vi "Sensirion SHT25 - VISA soft reset.vi"(8 "Error In":errorcluster, 11 "VISA in":refnum<visa-resource-name>) -> (0 "Error Out":errorcluster, 1 "readback":string, 3 "VISA out":refnum<visa-resource-name>)   [LabVIEW 2012]
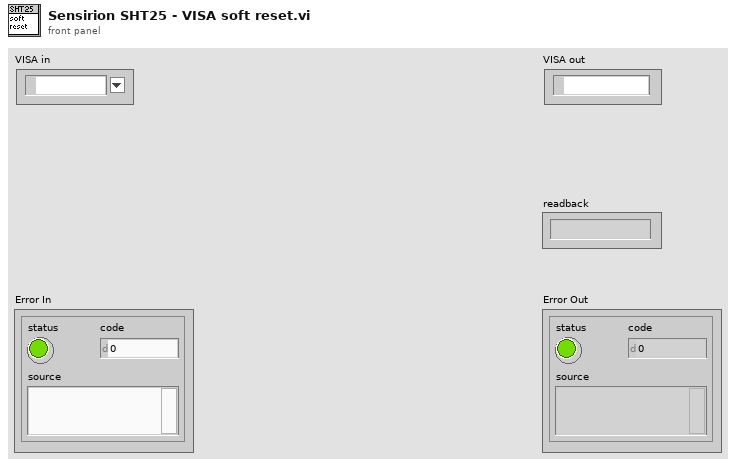
[diagram p1: front panel]
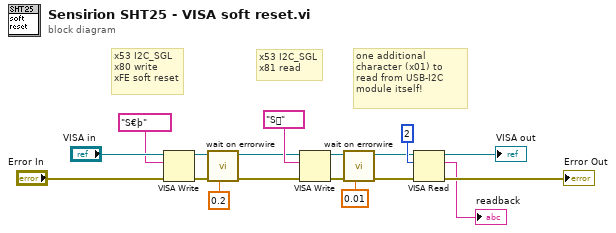
[diagram p0: block diagram]
diagram:
  # "one additional character (x01) to read from USB-I2C module itself!"
  # "x53 I2C_SGL\nx81 read"
  # "x53 I2C_SGL\nx80 write\nxFE soft reset"
  n1 = VISA Write(VISA resource name="VISA in", write buffer="S€þ", error in (no error)="Error In") -> (VISA resource name out=w9:refnum<visa-resource-name>, error out=w11:errorcluster)  [unwired: 1 out]
  n2 = call "wait on errorwire.vi"("Delay Time (s)"=0.2, "error in (no error)"=w11) -> ("error out"=w8:errorcluster)  [unwired: 9 in]
  n3 = VISA Write(VISA resource name=w9, write buffer="S", error in (no error)=w8) -> (VISA resource name out=w6:refnum<visa-resource-name>, error out=w4:errorcluster)  [unwired: 1 out]
  n4 = call "wait on errorwire.vi"("Delay Time (s)"=0.01, "error in (no error)"=w4) -> ("error out"=w3:errorcluster)  [unwired: 9 in]
  n5 = VISA Read(VISA resource name=w6, byte count=u32 2, error in (no error)=w3) -> (VISA resource name out=→"VISA out":refnum<visa-resource-name>, read buffer=→"readback":string, error out=→"Error Out":errorcluster)  [unwired: 1 out]
